vi "TCP Server Get Data.vi"(8 "error in (no error)":errorcluster, 11 "TCP Server":refnum<class "JKI TCP Server.lvclass">) -> (0 "error out":errorcluster, 2 "Data out":T1, 3 "TCP Server out":refnum<class "JKI TCP Server.lvclass">)   [LabVIEW 2020, in "JKI TCP Server.lvclass"]
doc: "Gets the GOOP data structure without mutex"
uses:
  JKI TCP Server.lvclass
  _Data Structures/TCP Server Data.ctl
  _Data Structures/TCP Server Listener Info Cluster.ctl
  _Data Structures/TCP Server Connection Info Cluster.ctl
  _Data Structures/TCP Server Handler RefNum.ctl
  _Data Structures/TCP Server Object Data Core Task Enum.ctl
  JKI TCP Server.lvclass/JKI TCP Server.ctl
panel:
  # "OpenGOOP Get Data.vi\n\nGets the GOOP data structure without mutex\n\nCopyright (C) 2002 Jim Kring jim@jimkring.com\n\nPlease visit http://www.OpenG.org to learn about the\nOpen Source LabVIEW software movement.\n\nThis library is free software; you can redistribute it and/or\nmodify it under the terms of the GNU Lesser General Public\nLicense as published by the Free Software Foundation; either\nversion 2.1 of the License, or (at your option) any later version.\nThis library is distributed in the hope that it will be useful,\nbut WITHOUT ANY WARRANTY; without even the implied warranty of\nMERCHANTABILITY or FITNESS FOR A PARTICULAR PURPOSE. See the GNU\nLesser General Public License for more details.\nYou should have received a copy of the GNU Lesser General Public\nLicense along with this library; if not, write to the Free Software\nFoundation, Inc., 59 Temple Place, Suite 330, Boston, MA 02111-1307 USA"
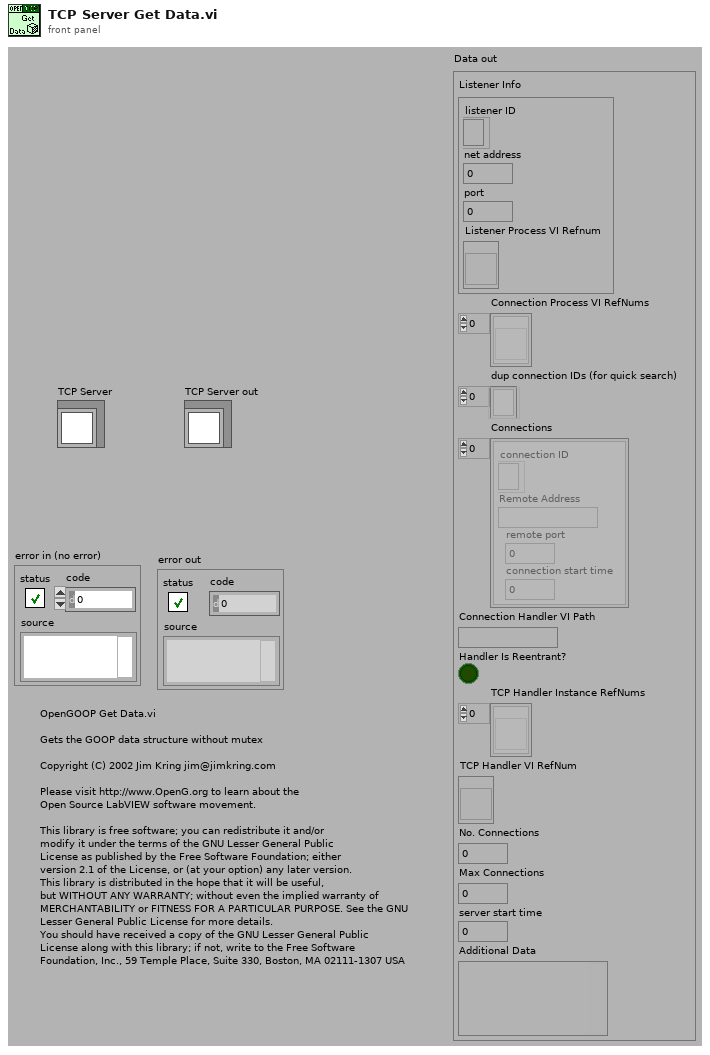
[diagram p1: front panel]
types:
  T1 = typedef "JKI TCP Server.lvclass/TCP Server Data.ctl" = cluster{"Listener Info":T2, "Connection Process VI RefNums":refnum<vi>[], "dup connection IDs (for quick search)":refnum<k5>[], "Connections":T3[], "Connection Handler VI Path":path, "Handler Is Reentrant?":bool, "TCP Handler Instance RefNums":T4[], "TCP Handler VI RefNum":T4, "No. Connections":u32, "Max Connections":u32, "server start time":u32, "Additional Data":variant}
  T2 = typedef "JKI TCP Server.lvclass/TCP Server Listener Info Cluster.ctl" = cluster{"listener ID":refnum<k5>, "net address":u32, "port":u16, "Listener Process VI Refnum":refnum<vi>}
  T3 = typedef "JKI TCP Server.lvclass/TCP Server Connection Info Cluster.ctl" = cluster{"connection ID":refnum<k5>, "Remote Address":string, "remote port":u16, "connection start time":u32}
  T4 = typedef "JKI TCP Server.lvclass/TCP Server Handler RefNum.ctl" = refnum<vi>
  T5 = typedef "JKI TCP Server.lvclass/TCP Server Object Data Core Task Enum.ctl" = enum16{"read", "write", "init"}
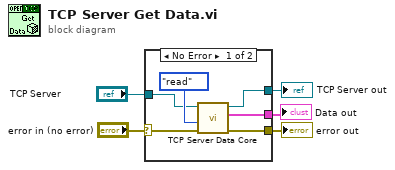
[diagram p0: block diagram]
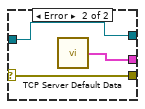
[diagram p2: hidden frame]
diagram:
  n1 = case shown="No Error" "error in (no error)" {
    selector: "error in (no error)" -> [w10 w14]
    tunnel: [w11 w14] -> w5
    tunnel: [w8 w13] -> w3
    tunnel: [w7 w12] -> w2
    tunnel: "TCP Server" -> [w6 w12]
    frame No Error {
      n2 = call "TCP Server Data Core.vi"("error in (no error)"=w10, "task (read)"=TCP_Server_Object_Data_Core_Task_Enum."read", "Refnum"=w6) -> ("error out"=w11:errorcluster, "Data out"=w8:T1, "dup Refnum"=w7:refnum<class "JKI TCP Server.lvclass">)  [unwired: 6 in]
    }
    frame Error {
      n3 = call "TCP Server Default Data.vi"() -> ("Data out"=w13:T1)
    }
  }
  "error out" <- w5
  "Data out" <- w3
  "TCP Server out" <- w2
